vi "Theta 2.vi"(5 "XYZ_60":dbl[](array[numeric])=[0.0, 0.0, 0.0], 7 "XYZ_0":dbl[](array[numeric])=[0.0, 0.0, 0.0], 10 "theta_0":dbl, 11 "6R Type 2 Serial Arm Class in":refnum<class "NI_Robotics_6R Type 2 Serial Arm Class.lvclass">) -> (1 "Valid":bool, 2 "theta_2 array":dbl[](array[numeric]), 3 "6R Type 2 Serial Arm Class out":refnum<class "NI_Robotics_6R Type 2 Serial Arm Class.lvclass">)   [LabVIEW 2017, in "NI_Robotics_6R Type 2 Serial Arm Class.lvclass"]
uses:
  <vilib>/robotics/Kinematics/Analytical/6R/Type 2/NI_Robotics_6R Type 2 Serial Arm Class.lvclass
  c:/Program Files (x86)/National Instruments/LabVIEW 2017/vi.lib/robotics/Kinematics/Analytical/Generic/NI_Robotics_Analytical Serial Arm Class.lvclass
  <vilib>/robotics/Kinematics/Link/NI_Robotics_Link.lvclass/NI_Robotics_Link.ctl
  <vilib>/robotics/Kinematics/Link/Get Kinematic Parameters.vi
  <vilib>/robotics/Kinematics/Analytical/Generic/NI_Robotics_Analytical Serial Arm Class.lvclass
  c:/Program Files (x86)/National Instruments/LabVIEW 2017/vi.lib/robotics/Kinematics/Robot/NI_Robotics_Serial Robot Arm.lvclass
  <vilib>/robotics/Kinematics/Analytical/Generic/Accessors/Read alpha_n0.vi
  <vilib>/robotics/Kinematics/Robot/Get Links.vi
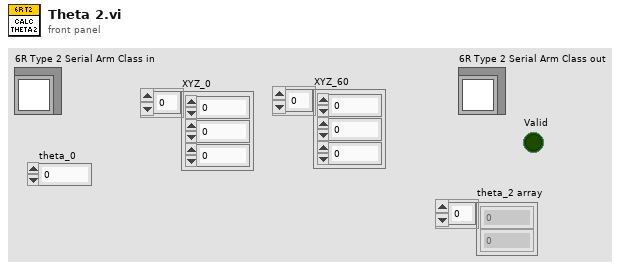
[diagram p1: front panel]
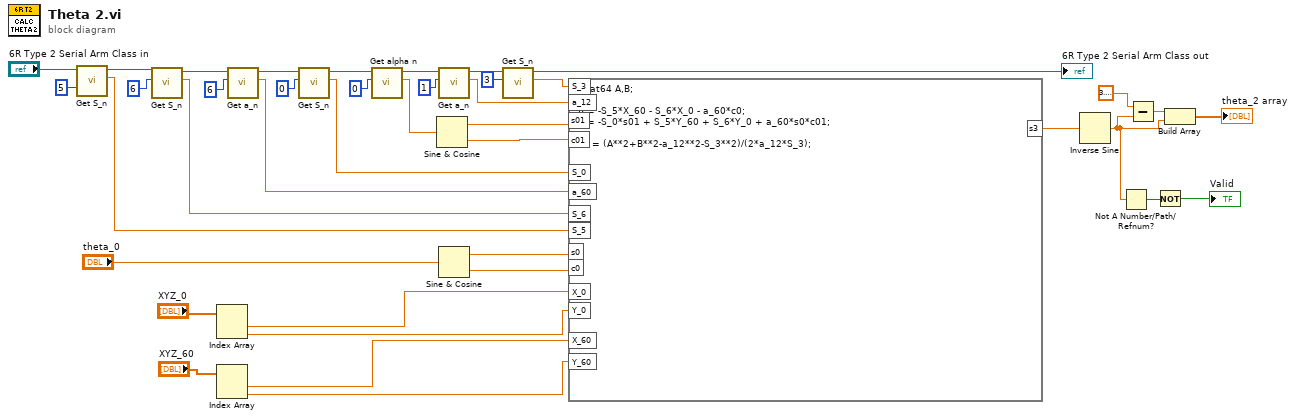
[diagram p0: block diagram]
diagram:
  n1 = call <vilib>:"Get S_n.vi"("n"=5, "Analytical Serial Arm Class in"="6R Type 2 Serial Arm Class in") -> ("S_n"=w24:dbl, "Analytical Serial Arm Class out"=w38:refnum<class "NI_Robotics_6R Type 2 Serial Arm Class.lvclass">)  [unwired: 8 in]
  n2 = call <vilib>:"Get S_n.vi"("n"=6, "Analytical Serial Arm Class in"=w38) -> ("S_n"=w25:dbl, "Analytical Serial Arm Class out"=w36:refnum<class "NI_Robotics_6R Type 2 Serial Arm Class.lvclass">)  [unwired: 8 in]
  n3 = Index Array(array="XYZ_0") -> (element #1=w18:dbl, element #2=w17:dbl)  [unwired: 2 in]
  n4 = Index Array(array="XYZ_60") -> (element #1=w15:dbl, element #2=w16:dbl)  [unwired: 2 in]
  n5 = call <vilib>:"Get a_n.vi"("n"=6, "Analytical Serial Arm Class in"=w36) -> ("a_n"=w26:dbl, "Analytical Serial Arm Class out"=w34:refnum<class "NI_Robotics_6R Type 2 Serial Arm Class.lvclass">)  [unwired: 8 in]
  n6 = call <vilib>:"Get S_n.vi"("n"=0, "Analytical Serial Arm Class in"=w34) -> ("S_n"=w27:dbl, "Analytical Serial Arm Class out"=w32:refnum<class "NI_Robotics_6R Type 2 Serial Arm Class.lvclass">)  [unwired: 8 in]
  n7 = call <vilib>:"Get alpha n.vi"("n"=0, "Analytical Serial Arm Class in"=w32) -> ("alpha n"=w30:dbl, "Analytical Serial Arm Class out"=w14:refnum<class "NI_Robotics_6R Type 2 Serial Arm Class.lvclass">)  [unwired: 8 in]
  n8 = Sine & Cosine(0:w30) -> (1:w29:dbl, 2:w28:dbl)
  n9 = call <vilib>:"Get a_n.vi"("n"=1, "Analytical Serial Arm Class in"=w14) -> ("a_n"=w8:dbl, "Analytical Serial Arm Class out"=w12:refnum<class "NI_Robotics_6R Type 2 Serial Arm Class.lvclass">)  [unwired: 8 in]
  n10 = Sine & Cosine(0:"theta_0") -> (1:w22:dbl, 2:w21:dbl)
  n11 = call <vilib>:"Get S_n.vi"("n"=3, "Analytical Serial Arm Class in"=w12) -> ("S_n"=w9:dbl, "Analytical Serial Arm Class out"=→"6R Type 2 Serial Arm Class out":refnum<class "NI_Robotics_6R Type 2 Serial Arm Class.lvclass">)  [unwired: 8 in]
  n12 = formula code="float64 A,B;\n\nA = -S_5*X_60 - S_6*X_0 - a_60*c0;\nB = -S_0*s01 + S_5*Y_60 + S_6*Y_0 + a_60*s0*c01;\n\ns3 = (A**2+B**2-a_12**2-S_3**2)/(2*a_12*S_3);"("s01"=w29, "c01"=w28, "S_0"=w27, "a_60"=w26, "S_6"=w25, "S_5"=w24, "s0"=w22, "c0"=w21, "X_0"=w18, "Y_0"=w17, "X_60"=w15, "Y_60"=w16, "S_3"=w9, "a_12"=w8) -> ("s3"=w7:dbl)
  n13 = Inverse Sine(1:w7) -> (0:w1:dbl)
  n14 = Not A Number/Path/Refnum?(number/path/refnum=w1) -> (NaN/Path/Refnum?=w3:bool)
  n15 = Subtract(x=3.141592653589793, y=w1) -> (x-y=w5:dbl)
  n16 = Not(x=w3) -> (.not. x?=→"Valid":bool)
  n17 = Build Array(w5, w1) -> (→"theta_2 array":dbl[])
